vi "COMTRADE List Private Contents.vi"(8 "error in (no error)":errorcluster, 10 "manufacturer name":string, 11 "task in":T1={"file refnums"=[], "Data Object"=refnum, "config info"={"station_name"="", "rec_dev_id"="", "rev_year"=1999.0, "TT"=0, "##A"=0, "##D"=0, "analog channel info"=[], "status channel info"=[], "lf"=50.0, "nrates"=0, "samp info"=[], "initial timestamp"=timestamp(0 s since 1904-01-01), "trigger timestamp"=timestamp(0 s since 1904-01-01), "ft"=enum."Binary", "timemult"=1.0}, "public inf content"={"Source"="", "Record Type"=enum."Unknown", "Phase ID"="", "Event Description"="", "Device ID"="", "Distance of Fault"=-1.0, "Distance Unit"=enum."Miles", "Max_Current"=inf, "Min_Current"=-inf, "Max_Voltage"=inf, "Min_Voltage"=-inf, "EventNoteCount"=0, "Event Information"=[]}, "private inf content"=[], "internal buffers"={"start index"=1, "config to public inf"=enum."disabled", "static config info"="", "static file_des record inf"="", "static file_des channel inf"="", "public inf"="", "private inf"=""}} {"public inf content"."Event Information"."min sample number" max=9999999999; "public inf content"."Event Information"."max sample number" max=9999999999; "config info"."nrates" max=999; "config info"."status channel info"."Dn" min=1 max=999999; "config info"."analog channel info"."An" min=1 max=999999; "config info"."trigger timestamp" format="%<%H:%M:%S%6u\n%d/%m/%Y>T"; "config info"."initial timestamp" format="%<%H:%M:%S%6u\n%d/%m/%Y>T"; "config info"."##D" max=999999; "config info"."##A" max=999999; "config info"."TT" min=1 max=999999; "config info"."rev_year" min=1999.0 max=1999.0}) -> (0 "error out":errorcluster, 1 "manufacturer/section names":string[][](array[string]), 2 "manufacturer names":string[](array[string]), 3 "task out":T1={"file refnums"=[], "Data Object"=refnum, "config info"={"station_name"="", "rec_dev_id"="", "rev_year"=1999.0, "TT"=0, "##A"=0, "##D"=0, "analog channel info"=[], "status channel info"=[], "lf"=50.0, "nrates"=0, "samp info"=[], "initial timestamp"=timestamp(0 s since 1904-01-01), "trigger timestamp"=timestamp(0 s since 1904-01-01), "ft"=enum."Binary", "timemult"=1.0}, "public inf content"={"Source"="", "Record Type"=enum."Unknown", "Phase ID"="", "Event Description"="", "Device ID"="", "Distance of Fault"=-1.0, "Distance Unit"=enum."Miles", "Max_Current"=inf, "Min_Current"=-inf, "Max_Voltage"=inf, "Min_Voltage"=-inf, "EventNoteCount"=0, "Event Information"=[]}, "private inf content"=[], "internal buffers"={"start index"=1, "config to public inf"=enum."disabled", "static config info"="", "static file_des record inf"="", "static file_des channel inf"="", "public inf"="", "private inf"=""}} {"public inf content"."Event Information"."min sample number" max=9999999999; "public inf content"."Event Information"."max sample number" max=9999999999; "config info"."nrates" max=999; "config info"."status channel info"."Dn" min=1 max=999999; "config info"."analog channel info"."An" min=1 max=999999; "config info"."trigger timestamp" format="%<%H:%M:%S%6u\n%d/%m/%Y>T"; "config info"."initial timestamp" format="%<%H:%M:%S%6u\n%d/%m/%Y>T"; "config info"."##D" max=999999; "config info"."##A" max=999999; "config info"."TT" min=1 max=999999; "config info"."rev_year" min=1999.0 max=1999.0})   [LabVIEW 2013, in "NI_EP_COMTRADE.lvlib"]
doc: "Lists all the section names of the specified manufacturer name. If <B>manufacturer name</B> is empty, this VI returns all the manufacturer names and section names. You must set <B>open mode</B> to Open (read only) in the COMTRADE Open VI to open the .hdr file. Otherwise this VI returns an error."
uses:
  <vilib>/addons/Electrical Power/File IO/NI_EP_COMTRADE.lvlib
  <vilib>/addons/Electrical Power/File IO/COMTRADE/typedefs/ep_Task.ctl
  <vilib>/addons/Electrical Power/File IO/COMTRADE/typedefs/ep_Config Info.ctl
  <vilib>/addons/Electrical Power/File IO/COMTRADE/typedefs/ep_Analog Channel Info.ctl
  <vilib>/addons/Electrical Power/File IO/COMTRADE/typedefs/ep_Status Channel Info.ctl
  <vilib>/addons/Electrical Power/File IO/COMTRADE/typedefs/ep_File Format.ctl
  <vilib>/addons/Electrical Power/File IO/COMTRADE/typedefs/ep_Public Inf Content.ctl
  <vilib>/addons/Electrical Power/File IO/COMTRADE/typedefs/ep_Public Event Inf.ctl
  <vilib>/addons/Electrical Power/File IO/COMTRADE/typedefs/ep_Private Inf Content.ctl
  <vilib>/Platform/storage/Storage.llb/Get Property (Storage Refnums).vi
  <vilib>/Platform/storage/Storage.llb/Get Property (I32).vi
  <vilib>/Platform/storage/Storage.llb/Get Property (String).vi
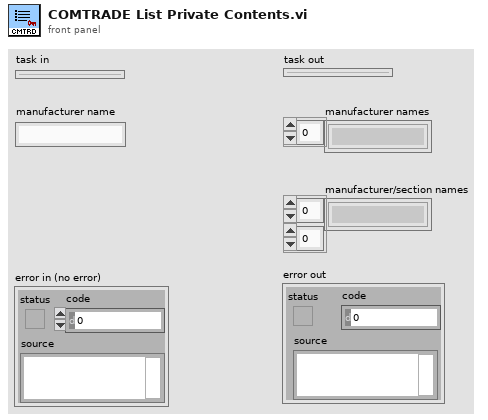
[diagram p1: front panel]
types:
  T1 = typedef "NI_EP_COMTRADE.lvlib/ep_Task.ctl" = cluster{"file refnums":refnum<file>[], "Data Object":refnum<k20>, "config info":T2, "public inf content":T6, "private inf content":T8, "internal buffers":cluster{"start index":u32, "config to public inf":enum16{"disabled", "enabled", "buffered"}, "static config info":string, "static file_des record inf":string, "static file_des channel inf":string, "public inf":string, "private inf":string}}
  T2 = typedef "NI_EP_COMTRADE.lvlib/ep_Config Info.ctl" = cluster{"station_name":string, "rec_dev_id":string, "rev_year":dbl, "TT":u32, "##A":u32, "##D":u32, "analog channel info":T3[], "status channel info":T4[], "lf":sgl, "nrates":u16, "samp info":cluster{"samp":sgl, "endsamp":u32}[], "initial timestamp":timestamp, "trigger timestamp":timestamp, "ft":T5, "timemult":sgl}
  T3 = typedef "NI_EP_COMTRADE.lvlib/ep_Analog Channel Info.ctl" = cluster{"An":u32, "ch_id":string, "ph":string, "ccbm":string, "uu":string, "a":sgl, "b":sgl, "skew":sgl, "min":i32, "max":i32, "primary":sgl, "secondary":sgl, "PS":enum16{"P", "S"}}
  T4 = typedef "NI_EP_COMTRADE.lvlib/ep_Status Channel Info.ctl" = cluster{"Dn":u32, "ch_id":string, "ph":string, "ccbm":string, "Y":bool}
  T5 = typedef "NI_EP_COMTRADE.lvlib/ep_File Format.ctl" = enum16{"ASCII", "Binary"}
  T6 = typedef "NI_EP_COMTRADE.lvlib/ep_Public Inf Content.ctl" = cluster{"Source":string, "Record Type":enum16{"Fault", "Unknown", "Misoperation", "Close", "Trip", "Reclose", "Power swing", "Simulation"}, "Phase ID":string, "Event Description":string, "Device ID":string, "Distance of Fault":dbl, "Distance Unit":enum16{"Miles", "Kilometers", "Percent of line", "Percent of setting", "Ohms"}, "Max_Current":dbl, "Min_Current":dbl, "Max_Voltage":dbl, "Min_Voltage":dbl, "EventNoteCount":u32, "Event Information":T7[]}
  T7 = typedef "NI_EP_COMTRADE.lvlib/ep_Public Event Inf.ctl" = cluster{"channel number":u32, "max value":dbl, "min value":dbl, "max sample number":u64, "min sample number":u64, "max sample text":string[], "min sample text":string[]}
  T8 = typedef "NI_EP_COMTRADE.lvlib/ep_Private Inf Content.ctl" = cluster{"Section Header":string, "Entry Names":string[], "Entry Values":string[]}[]
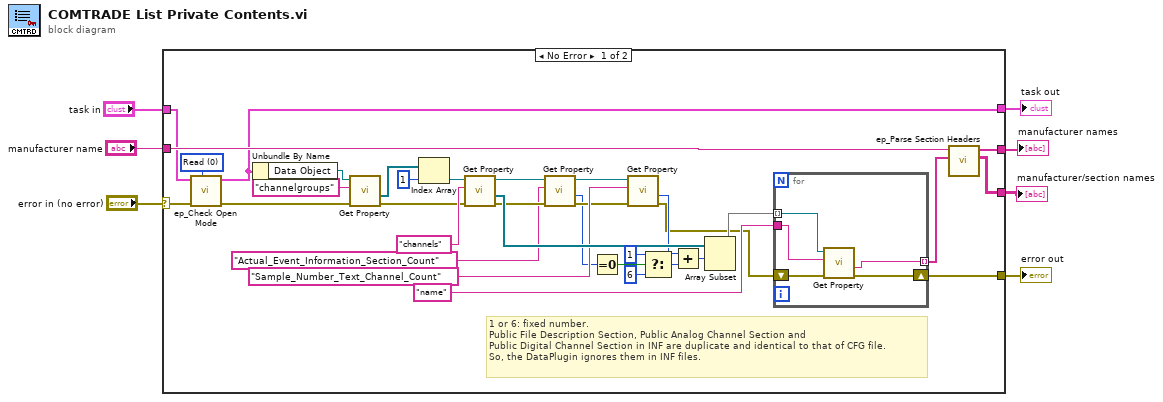
[diagram p0: block diagram]
diagram:
  n1 = case shown="No Error" "error in (no error)" {
    selector: "error in (no error)" -> [w11 w47]
    tunnel: "task in" -> [w9 w48]
    tunnel: [w8 w48] -> w3
    tunnel: [w27 w47] -> w6
    tunnel: "manufacturer name" -> [w16 _]
    tunnel: [w14 _] -> w2
    tunnel: [w13 _] -> w1
    frame No Error {
      w12 = u16 0 items=["Read", "Write"] ("file type")
      # "1 or 6: fixed number.\nPublic File Description Section, Public Analog Channel Section and \nPublic Digital Channel Section in INF are duplicate and identical to that of CFG file. \nSo, the DataPlugin ignores them in INF files."
      n2 = call <vilib>:"ep_Check Open Mode.vi"("expected mode"=w12, "error in (no error)"=w11, "task in"=w9) -> ("error out"=w10:errorcluster, "task out"=w8:T1)  [unwired: 7 in]
      n3 = Unbundle By Name(w8) -> ("Data Object"=w41:refnum<k20>)
      n4 = call-poly <vilib>:"Get Property.vi"("error in (no error)"=w10, "Property name"="channelgroups", "storage refnum"=w41) -> ("error out"=w31:errorcluster, "Value"=w40:refnum<k20>[])  [unwired: 6 in, 1 out]
      n5 = Index Array(array=w40, index=1) -> (element=w36:refnum<k20>)
      n6 = call-poly <vilib>:"Get Property.vi"("error in (no error)"=w31, "Property name"="channels", "storage refnum"=w36) -> ("error out"=w26:errorcluster, "Value"=w35:refnum<k20>[], "storage refnum out"=w18:refnum<k20>)  [unwired: 6 in]
      n7 = call-poly <vilib>:"Get Property.vi"("error in (no error)"=w26, "Property name"="Actual_Event_Information_Section_Count", "storage refnum"=w18) -> ("error out"=w25:errorcluster, "Value"=w22:i32, "storage refnum out"=w17:refnum<k20>)  [unwired: 6 in]
      n8 = Equal To 0?(x=w22) -> (x = 0?=w23:bool)
      n9 = call-poly <vilib>:"Get Property.vi"("error in (no error)"=w25, "Property name"="Sample_Number_Text_Channel_Count", "storage refnum"=w17) -> ("error out"=w28:errorcluster, "Value"=w33:i32)  [unwired: 6 in, 1 out]
      n10 = Select(t=1 ("index"), s=w23, f=6 ("index")) -> (s? t:f=w21:i32)
      n11 = Add(x=w33, y=w21) -> (x+y=w34:i32)
      n12 = Array Subset(array=w35, index=w34) -> (w30:refnum<k20>[])  [unwired: 1 in]
      n13 = for {
        tunnel: w30 -> [w46] mode=indexing
        tunnel: "name" ("Property name") -> [w45]
        shift-right: [w43] -> w27
        shift-left: w28 -> [w42]
        tunnel: [w44] -> w15 mode=indexing
        n14 = call-poly <vilib>:"Get Property.vi"("error in (no error)"=w42, "Property name"=w45, "storage refnum"=w46) -> ("error out"=w43:errorcluster, "Value"=w44:string)  [unwired: 6 in, 1 out]
      }
      n15 = call <vilib>:"ep_Parse Section Headers.vi"("raw section headers"=w15, "manufacturer name"=w16) -> ("manufacturer/section names"=w13:string[][], "manufacturer names"=w14:string[])  [unwired: 8 in]
    }
    frame Error {
    }
  }
  "error out" <- w6
  "task out" <- w3
  "manufacturer names" <- w2
  "manufacturer/section names" <- w1
